vi "ErrorDescr.vi"(11 "ErrorCode":i32) -> (3 "Desc":string)   [LabVIEW 2017]
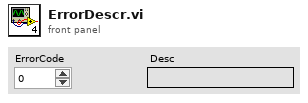
[diagram p1: front panel]
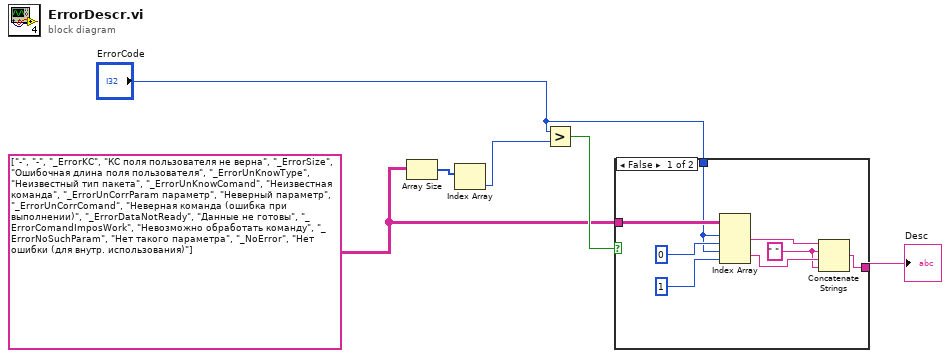
[diagram p0: block diagram]
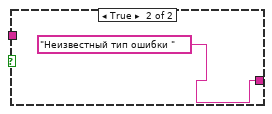
[diagram p2: hidden frame]
diagram:
  w2 = string[][] [["-", "-"], ["_ErrorKC", "КС поля пользователя не верна"], ["_ErrorSize", "Ошибочная длина поля пользователя"], ["_ErrorUnKnowType", "Неизвестный тип пакета"], ["_ErrorUnKnowComand", "Неизвестная команда"], ["_ErrorUnCorrParam параметр", "Неверный параметр"], ["_ErrorUnCorrComand", "Неверная команда (ошибка при выполнении)"], ["_ErrorDataNotReady", "Данные не готовы"], ["_ErrorComandImposWork", "Невозможно обработать команду"], ["_ErrorNoSuchParam", "Нет такого параметра"], ["_NoError", "Нет ошибки (для внутр. использования)"]]
  n1 = Array Size(array=w2) -> (size(s)=w3:i32[])
  n2 = Index Array(array=w3) -> (element=w4:i32)  [unwired: 1 in]
  n3 = Greater?(x="ErrorCode", y=w4) -> (0:w5:bool)
  n4 = case shown="False" w5 {
    tunnel: [w10 "Неизвестный тип ошибки "] -> w1
    tunnel: w2 -> [w8 _]
    tunnel: "ErrorCode" -> [w7 _]
    frame False {
      w9 = " " ("string")
      n5 = Index Array(array=w8, index (row) #1=w7, index (col) #1=0 ("disabled index (col)"), index (row) #2=w7, index (col) #2=1 ("disabled index (col)")) -> (element #1=w12:string, element #2=w11:string)
      n6 = Concatenate Strings(w12, w9, w11, w9) -> (w10:string)
    }
    frame True {
    }
  }
  "Desc" <- w1
